vi "DSF.Transceiver.UDP.Set Tx Parameters.vi"(10 "Tx parameters":T1[](array[typedef]) {"address" format="%.0x"}, 11 "DSF.Transceiver.UDP in":refnum<class "DSF.Transceiver.UDP.lvclass">) -> (3 "DSF.Transceiver.UDP out":refnum<class "DSF.Transceiver.UDP.lvclass">)   [LabVIEW 2017, in "DSF.Transceiver.UDP.lvlib" / "DSF.Transceiver.UDP.lvclass"]
uses:
  DSF.Transceiver.UDP.lvclass
  DSF.Transceiver.UDP.Tx Parameters.ctl
  DSF.Transceiver.UDP.lvclass/DSF.Transceiver.UDP.ctl
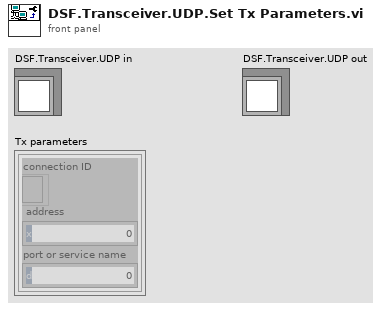
[diagram p1: front panel]
types:
  T1 = typedef "DSF.Transceiver.UDP.lvlib/DSF.Transceiver.UDP.lvclass/DSF.Transceiver.UDP.Tx Parameters.ctl" = cluster{"connection ID":refnum<k16>, "address":u32, "port or service name":u16}
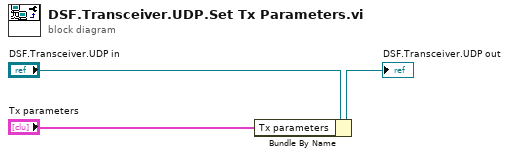
[diagram p0: block diagram]
diagram:
  n1 = Bundle By Name(cluster="DSF.Transceiver.UDP in", "Tx parameters"="Tx parameters") -> (→"DSF.Transceiver.UDP out":refnum<class "DSF.Transceiver.UDP.lvclass">)
